vi "AppendCommandsToStep.vi"(10 "CommandsToAppend":string[](array[string])) -> ()   [LabVIEW 2016]
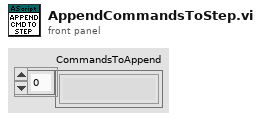
[diagram p1: front panel]
types:
  T1 = cluster{"Return Variable Names":refnum<vi>, "ArgumentsBox":refnum<vi>, "Routine":refnum<vi>, "AddCmd":refnum<vi>, "ClearSteps":refnum<vi>, "AddStep":refnum<vi>, "DeleteAuto":refnum<vi>, "DeleteCommand":refnum<vi>, "DeleteStep":refnum<vi>, "TemplateOpen":refnum<vi>, "SaveStep":refnum<vi>, "LoadAuto":refnum<vi>, "SaveAuto":refnum<vi>, "LoadStep":refnum<vi>, "AutoFiles":refnum<vi>, "DeleteLog":refnum<vi>, "GetLogFile":refnum<vi>, "Auto Script on Robot":refnum<vi>, "DLfromRIO":refnum<vi>, "Autoscript Layout":refnum<vi>, "Auto Script Name":refnum<vi>, "ULtoRIO":refnum<vi>}
  T2 = cluster{"Number":i32, "Name":string, "Commands":string[], "WaitForExecution":bool}[]
  T3 = cluster{"Number":i32, "Name":string, "Commands":string[], "WaitForExecution":bool}
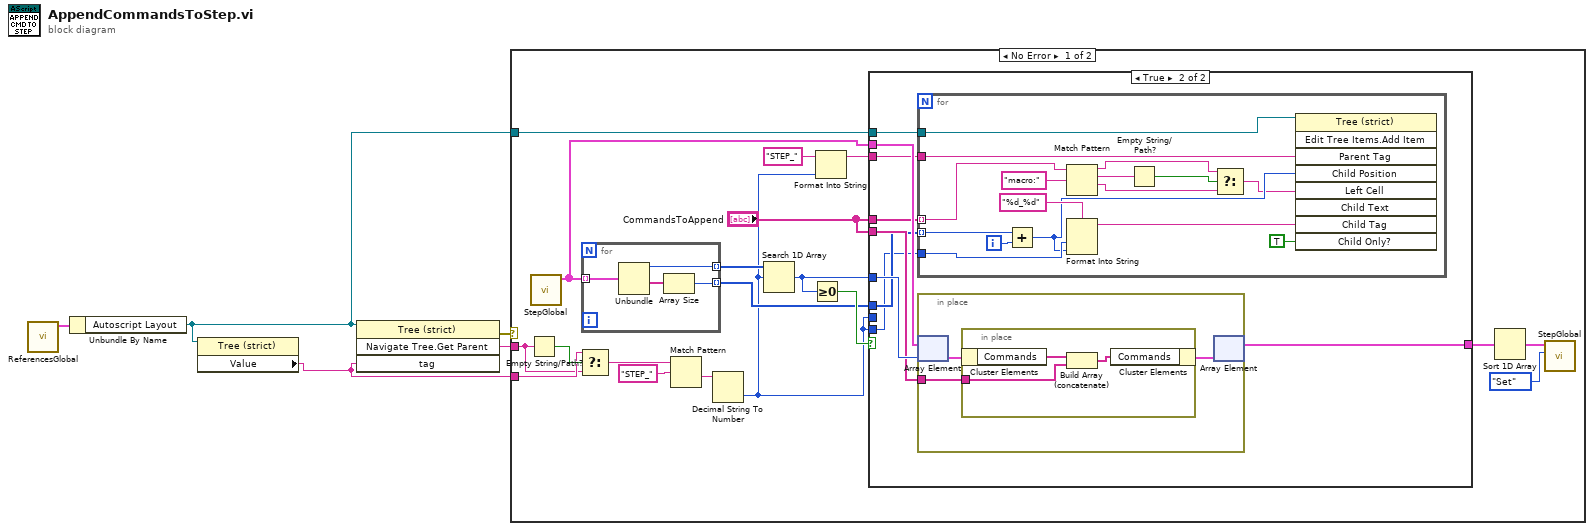
[diagram p0: block diagram]
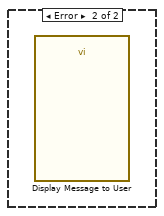
[diagram p3: hidden frame]
diagram:
  n1 = call "ReferencesGlobal.vi"() -> ("AscriptRefsOut"=w3:T1)  [unwired: 11 in]
  n2 = Unbundle By Name(w3) -> ("Autoscript Layout"=w5:refnum<vi>)
  n3 = property class="Tree (strict)"(reference=w5) -> ("Value"=w1:string)  [unwired: 1 in, 2 out]
  n4 = invoke class="Tree (strict)" method="Navigate Tree.Get Parent"(reference=w5, "tag"=w1) -> (error out=w2:errorcluster, "Navigate Tree:Get Parent"=w4:string)  [unwired: 2 in, 2 out]
  n5 = case shown="No Error" w2 {
    tunnel: w5 -> [w16 _]
    tunnel: w1 -> [w14 _]
    tunnel: w4 -> [w13 _]
    frame No Error {
      n6 = Empty String/Path?(string/path=w13) -> (empty?=w15:bool)
      n7 = call "StepGlobal.vi"() -> ("AutoScriptSteps out"=w8:T2)  [unwired: 11 in]
      n8 = Select(t=w14, s=w15, f=w13) -> (s? t:f=w12:string)
      n9 = for {
        tunnel: w8 -> [w60] mode=indexing
        tunnel: [w59] -> w24 mode=indexing
        tunnel: [w57] -> w19 mode=indexing
        n10 = Unbundle(w60) -> ("Number"=w59:i32, "Commands"=w58:string[])  [unwired: 2 out]
        n11 = Array Size(array=w58) -> (size(s)=w57:i32)
      }
      n12 = Match Pattern(string=w12, regular expression="STEP_") -> (after substring=w10:string)  [unwired: 1 in, 3 out]
      n13 = Decimal String To Number(string=w10) -> (number=w9:i32)  [unwired: 2 in, 1 out]
      n14 = Search 1D Array(1D array=w24, element=w9) -> (index of element=w22:i32)  [unwired: 1 in]
      n15 = Greater Or Equal To 0?(x=w22) -> (x >= 0?=w23:bool)
      n16 = Format Into String(initial string="STEP_", w9) -> (resulting string=w17:string)  [unwired: 2 in, 1 out]
      n17 = case shown="True" w23 {
        tunnel: w8 -> [w25 w34]
        tunnel: w22 -> [_ w33]
        tunnel: "CommandsToAppend" -> [_ w32]
        tunnel: [w25 w31] -> w21
        tunnel: w9 -> [_ _]
        tunnel: "CommandsToAppend" -> [_ w30]
        tunnel: w16 -> [_ w29]
        tunnel: w19 -> [_ w28]
        tunnel: w17 -> [_ w27]
        tunnel: w9 -> [_ w26]
        frame False {
        }
        frame True {
          n18 = for {
            tunnel: w30 -> [w42] mode=indexing
            tunnel: w29 -> [w50]
            tunnel: w28 -> [w35] mode=indexing
            tunnel: w27 -> [w48]
            tunnel: w26 -> [w46]
            i -> [w49]
            n19 = Add(x=w35, y=w49) -> (x+y=w45:i32)
            n20 = Match Pattern(string=w42, regular expression="macro:") -> (before substring=w38:string, match substring=w40:string, after substring=w37:string)  [unwired: 1 in, 1 out]
            n21 = Format Into String(format string="%d_%d", w46, w45) -> (resulting string=w44:string)  [unwired: 2 in, 1 out]
            n22 = Empty String/Path?(string/path=w40) -> (empty?=w39:bool)
            n23 = Select(t=w38, s=w39, f=w37) -> (s? t:f=w36:string)
            n24 = invoke class="Tree (strict)" method="Edit Tree Items.Add Item"(reference=w50, "Parent Tag"=w48, "Child Position"=w45, "Left Cell"=w36, "Child Tag"=w44, "Child Only?"=TRUE) -> ()  [unwired: 3 in, 9 out]
          }
          n25 = in-place {
            in-place-border: w32 -> [w51]
            n26 = in-place-array #1(w34, w33) -> (w53:T3)
            n27 = in-place {
              in-place-border: w51 -> [w54]
              n28 = in-place-cluster #2(w53) -> ("Commands"=w56:string[])
              n29 = Build Array (concatenate)(w56, w54) -> (w55:string[])
              n30 = in-place-cluster #2("Commands"=w55) -> (w52:T3)
            }
            n31 = in-place-array #1(w52) -> (w31:T2)  [unwired: 1 out]
          }
        }
      }
      n32 = Sort 1D Array(array=w21) -> (sorted array=w7:T2)
      n33 = call "StepGlobal.vi"("Action (Get)"=enum16{"Clear", "Append", "Set", "Get"}."Set", "AutoScriptSteps in"=w7) -> ()  [unwired: 9 in, 1 out]
    }
    frame Error {
      n34 = call "Display Message to User"() -> ()  [unwired: 10 in, 2 out]
    }
  }
